vi "F3Machine_2.vi"   [LabVIEW 2011]
uses:
  API/API DYM.lvlib
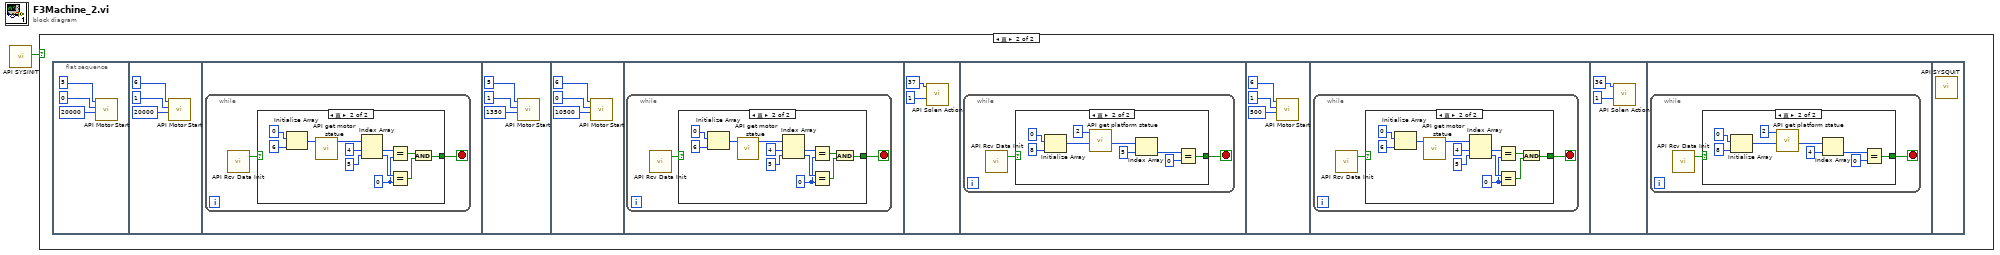
[diagram p0: block diagram]
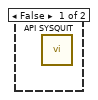
[diagram p2: hidden frame]
diagram:
  n1 = call "API SYSINIT.vi"() -> ("SYSINIT return value"=w1:bool)  [unwired: 11 in]
  n2 = case shown="真" w1 {
    frame False {
      n3 = call "API SYSQUIT.vi"() -> ()  [unwired: 12 in]
    }
    frame True {
      n4 = flat-sequence {
        frame #0 {
          n5 = call "API Motor Start.vi"("stepNum"=20000, "direction"=0, "motorNum"=5) -> ()  [unwired: 8 in, 1 out]
        }
        frame #1 {
          n6 = call "API Motor Start.vi"("stepNum"=20000, "direction"=1, "motorNum"=6) -> ()  [unwired: 8 in, 1 out]
        }
        frame #2 {
          n7 = while {
            stop <- w8 stop-if-true
            n8 = call "API Rcv Data Init.vi"() -> ("RTV"=w9:bool)  [unwired: 2 in, 1 out]
            n9 = case shown="真" w9 {
              selector: w9 -> [w10 _]
              tunnel: [w10 w11] -> w8
              frame False {
              }
              frame True {
                w14 = 0
                n10 = Initialize Array(0 ("元素"), 6 ("维数大小")) -> (w19:i32[])
                n11 = call "API get motor statue.vi"("motor statue array input"=w19) -> ("motor statue array output"=w18:i32[])  [unwired: 9 in, 1 out]
                n12 = Index Array(array=w18, index #1=4 ("索引"), index #2=5 ("索引")) -> (element #1=w16:i32, element #2=w15:i32)
                n13 = Equal?(x=w16, y=w14) -> (x = y?=w13:bool)
                n14 = Equal?(x=w15, y=w14) -> (x = y?=w12:bool)
                n15 = And(x=w13, y=w12) -> (x .and. y?=w11:bool)
              }
            }
          }
        }
        frame #3 {
          n16 = call "API Motor Start.vi"("stepNum"=1350, "direction"=1, "motorNum"=5) -> ()  [unwired: 8 in, 1 out]
        }
        frame #4 {
          n17 = call "API Motor Start.vi"("stepNum"=10500, "direction"=0, "motorNum"=6) -> ()  [unwired: 8 in, 1 out]
        }
        frame #5 {
          n18 = while {
            stop <- w29 stop-if-true
            n19 = call "API Rcv Data Init.vi"() -> ("RTV"=w30:bool)  [unwired: 2 in, 1 out]
            n20 = case shown="真" w30 {
              selector: w30 -> [w31 _]
              tunnel: [w31 w32] -> w29
              frame False {
              }
              frame True {
                w35 = 0
                n21 = Initialize Array(0 ("元素"), 6 ("维数大小")) -> (w40:i32[])
                n22 = call "API get motor statue.vi"("motor statue array input"=w40) -> ("motor statue array output"=w39:i32[])  [unwired: 9 in, 1 out]
                n23 = Index Array(array=w39, index #1=4 ("索引"), index #2=5 ("索引")) -> (element #1=w37:i32, element #2=w36:i32)
                n24 = Equal?(x=w37, y=w35) -> (x = y?=w34:bool)
                n25 = Equal?(x=w36, y=w35) -> (x = y?=w33:bool)
                n26 = And(x=w34, y=w33) -> (x .and. y?=w32:bool)
              }
            }
          }
        }
        frame #6 {
          n27 = call "API Solen Action.vi"("statue"=1, "solenNum"=37) -> ()  [unwired: 9 in, 1 out]
        }
        frame #7 {
          n28 = while {
            stop <- w46 stop-if-true
            n29 = call "API Rcv Data Init.vi"() -> ("RTV"=w47:bool)  [unwired: 2 in, 1 out]
            n30 = case shown="真" w47 {
              selector: w47 -> [w48 _]
              tunnel: [w48 w49] -> w46
              frame False {
              }
              frame True {
                n31 = Initialize Array(0 ("元素"), 8 ("维数大小")) -> (w54:i32[])
                n32 = call "API get platform statue.vi"("platformStatue input"=w54, "PlatformNum"=2) -> ("platformStatue output"=w53:i32[])  [unwired: 8 in, 1 out]
                n33 = Index Array(array=w53, index=5 ("索引")) -> (element=w51:i32)
                n34 = Equal?(x=w51, y=0) -> (x = y?=w49:bool)
              }
            }
          }
        }
        frame #8 {
          n35 = call "API Motor Start.vi"("stepNum"=500, "direction"=1, "motorNum"=6) -> ()  [unwired: 8 in, 1 out]
        }
        frame #9 {
          n36 = while {
            stop <- w61 stop-if-true
            n37 = call "API Rcv Data Init.vi"() -> ("RTV"=w62:bool)  [unwired: 2 in, 1 out]
            n38 = case shown="真" w62 {
              selector: w62 -> [w63 _]
              tunnel: [w63 w64] -> w61
              frame False {
              }
              frame True {
                w67 = 0
                n39 = Initialize Array(0 ("元素"), 6 ("维数大小")) -> (w72:i32[])
                n40 = call "API get motor statue.vi"("motor statue array input"=w72) -> ("motor statue array output"=w71:i32[])  [unwired: 9 in, 1 out]
                n41 = Index Array(array=w71, index #1=4 ("索引"), index #2=5 ("索引")) -> (element #1=w69:i32, element #2=w68:i32)
                n42 = Equal?(x=w69, y=w67) -> (x = y?=w66:bool)
                n43 = Equal?(x=w68, y=w67) -> (x = y?=w65:bool)
                n44 = And(x=w66, y=w65) -> (x .and. y?=w64:bool)
              }
            }
          }
        }
        frame #10 {
          n45 = call "API Solen Action.vi"("statue"=1, "solenNum"=36) -> ()  [unwired: 9 in, 1 out]
        }
        frame #11 {
          n46 = while {
            stop <- w78 stop-if-true
            n47 = call "API Rcv Data Init.vi"() -> ("RTV"=w79:bool)  [unwired: 2 in, 1 out]
            n48 = case shown="真" w79 {
              selector: w79 -> [w80 _]
              tunnel: [w80 w81] -> w78
              frame False {
              }
              frame True {
                n49 = Initialize Array(0 ("元素"), 8 ("维数大小")) -> (w86:i32[])
                n50 = call "API get platform statue.vi"("platformStatue input"=w86, "PlatformNum"=2) -> ("platformStatue output"=w85:i32[])  [unwired: 8 in, 1 out]
                n51 = Index Array(array=w85, index=4 ("索引")) -> (element=w83:i32)
                n52 = Equal?(x=w83, y=0) -> (x = y?=w81:bool)
              }
            }
          }
        }
        frame #12 {
          n53 = call "API SYSQUIT.vi"() -> ()  [unwired: 12 in]
        }
      }
    }
  }
